vi "acquire Sub Frame LV.vi"(8 "error in (no error)":errorcluster, 11 "expTime":sgl) -> (0 "error out":errorcluster)   [LabVIEW 2016, in "cameraLibrary.lvlib"]
doc: "Acquire frames continuously on the specified sub-window.\n\n\n\nvoid CAMERALIBRARYSHARED_EXPORT acquireSubFrameLV(float expTime);"
uses:
  cameraLibrary.lvlib
  cameraLibrary.dll
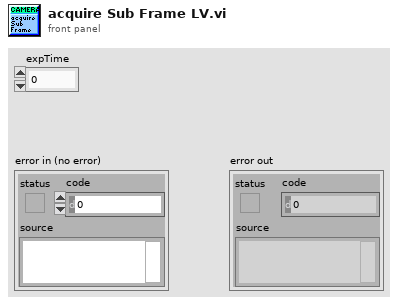
[diagram p1: front panel]
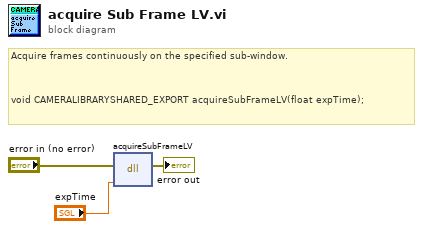
[diagram p0: block diagram]
diagram:
  # "Acquire frames continuously on the specified sub-window.\n\n\n\nvoid CAMERALIBRARYSHARED_EXPORT acquireSubFrameLV(float expTime);"
  n1 = dll-call lib="C:/Users/TMM/repos/EXPRES/FEM/FTT/support/Camera Library/cameraLibrary.*" fn="acquireSubFrameLV"(error in="error in (no error)", "expTime"="expTime") -> (error out=→"error out":errorcluster)  [unwired: 4 in, 1 out]
